vi "Remove Subscriber.vi"(8 "error in (no error)":errorcluster, 10 "Publisher to Remove":string, 11 "CIF_DAQ_DVR_Multi in":refnum<class "CIF_DAQ_DVR_Multi.lvclass">) -> (0 "error out":errorcluster, 3 "CIF_DAQ_DVR_Multi out":refnum<class "CIF_DAQ_DVR_Multi.lvclass">)   [LabVIEW 2021, in "CIF_DAQ_DVR_Multi.lvclass"]
uses:
  CIF_DAQ_DVR_Multi.lvclass
  CIF_DAQ_DVR_Multi.lvclass/CIF_DAQ_DVR_Multi.ctl
  ChannelCommon/typedef/Errors.ctl
  ChannelCommon/ChannelCommon.lvlib
  FIFO_DAQ_DVR/CIF_NIChn_FIFO_DAQ_DVR.lvclass
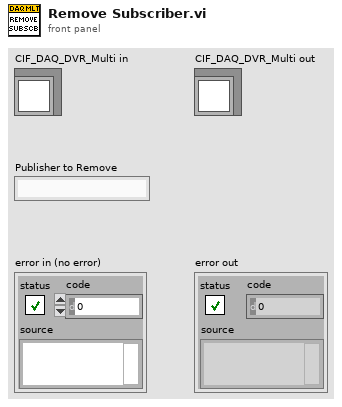
[diagram p1: front panel]
types:
  T1 = typedef "ChannelCommon.lvlib/Errors.ctl" = enum16{"gRPC Server Not Found", "Duplicate Channel", "Missing Channel", "Incorrect Type", "Flatten Error", "Unflatten Data", "Channel Length", "Plugin Connection", "gRPC Server Connection", "FIFO Unflatten", "Required Override", "Remove Not Found"}
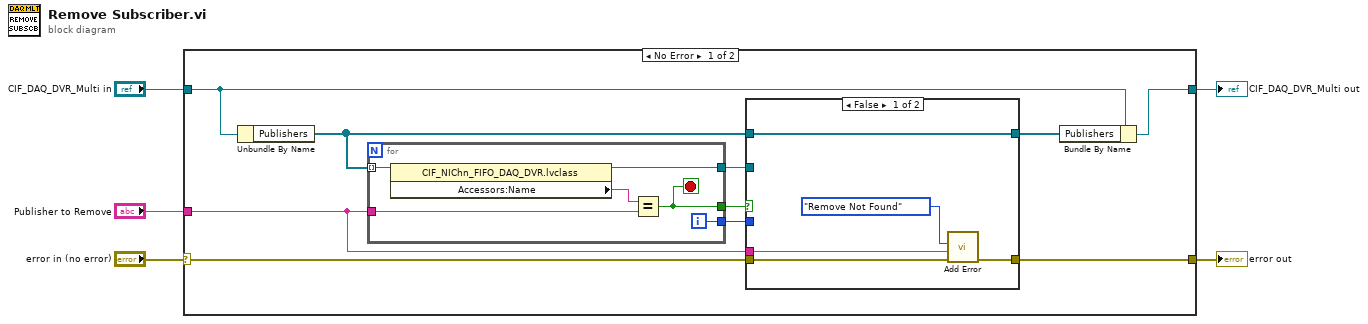
[diagram p0: block diagram]
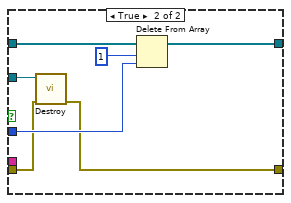
[diagram p2: hidden frame]
diagram:
  n1 = case shown="No Error" "error in (no error)" {
    selector: "error in (no error)" -> [w7 w35]
    tunnel: [w8 w35] -> w4
    tunnel: [w14 w34] -> w2
    tunnel: "CIF_DAQ_DVR_Multi in" -> [w15 w34]
    tunnel: "Publisher to Remove" -> [w6 _]
    frame No Error {
      n2 = Unbundle By Name(w15) -> ("Publishers"=w10:refnum<class "CIF_NIChn_FIFO_DAQ_DVR.lvclass">[])
      n3 = for {
        tunnel: w10 -> [w33] mode=indexing
        tunnel: w6 -> [w31]
        tunnel: [w30] -> w13
        tunnel: [w29] -> w12
        tunnel: [w28] -> w11
        i -> [w28]
        stop <- w29 stop-if-true
        n4 = property class="CIF_NIChn_FIFO_DAQ_DVR.lvclass"(reference=w33) -> (reference out=w30:refnum<class "CIF_NIChn_FIFO_DAQ_DVR.lvclass">, "Accessors:Name"=w32:string)  [unwired: 1 in, 1 out]
        n5 = Equal?(x=w32, y=w31) -> (x = y?=w29:bool)
      }
      n6 = case shown="False" w12 {
        tunnel: w10 -> [w20 w27]
        tunnel: w13 -> [_ w26]
        tunnel: w11 -> [_ w25]
        tunnel: w7 -> [w19 w23]
        tunnel: [w18 w22] -> w8
        tunnel: [w20 w21] -> w9
        tunnel: w6 -> [w16 _]
        frame False {
          n7 = call "Add Error.vi"("error in (no error)"=w19, "String to Append"=w16, "Error"=Errors."Remove Not Found") -> ("error out"=w18:errorcluster)  [unwired: 8 in]
        }
        frame True {
          n8 = call-dynamic "Destroy.vi"("error in (no error)"=w23, "CIF_NIChn_FIFO_DAQ in"=w26) -> ("error out"=w22:errorcluster)  [unwired: 8 in, 1 out]
          n9 = Delete From Array(array=w27, length=1, index=w25) -> (array with subset deleted=w21:refnum<class "CIF_NIChn_FIFO_DAQ_DVR.lvclass">[])  [unwired: 1 out]
        }
      }
      n10 = Bundle By Name(cluster=w15, "Publishers"=w9) -> (w14:refnum<class "CIF_DAQ_DVR_Multi.lvclass">)
    }
    frame Error {
    }
  }
  "error out" <- w4
  "CIF_DAQ_DVR_Multi out" <- w2
